vi "Close VISA.vi"   [LabVIEW 2009]
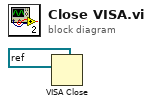
[diagram p0: block diagram]
diagram:
  n1 = VISA Close(VISA resource name=refnum<visa-resource-name> "COM1") -> ()  [unwired: 1 in, 1 out]
